vi "Get_modify_set_Protocol2.vi"() -> ()   [LabVIEW 2019]
uses:
  <vilib>/NI VeriStand/Custom Device API/Custom Device Item Ref.ctl
  Addon/Support Libraries/Protocols.lvlibp/TCP/TCP.lvclass
  C:/Dev/niveristand-instrument-addon-custom-device/Source/Addon/Support Libraries/Protocols.lvlibp/Protocol Parent/Protocol Parent.lvclass
  Scripting API/Scripting API.lvlib
  <vilib>/NI VeriStand/Custom Device API/Custom Device API.lvlib
panel:
  out "Instrument Addon Refnum Out":T1=18446744073709551615 format="%.0x"
  out "Error Out":errorcluster
  in  "Error In":errorcluster
  in  "Instrument Addon Refnum In":T1=18446744073709551615 format="%.0x"
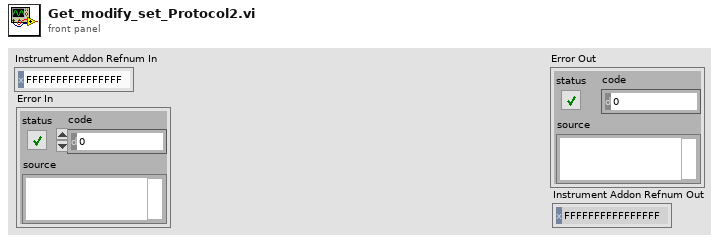
[diagram p1: front panel]
types:
  T1 = typedef "Custom Device API.lvlib/Custom Device Item Ref.ctl" = u64
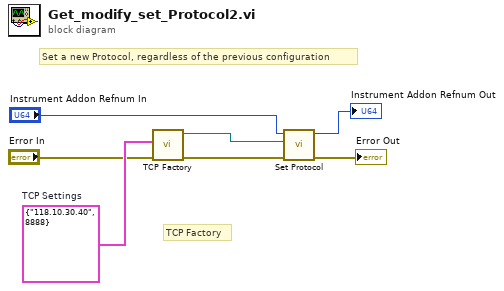
[diagram p0: block diagram]
diagram:
  w5 = cluster{"IP Address":string, "Port":u16} {"IP Address"="118.10.30.40", "Port"=8888}  # TCP Settings
  # "TCP Factory"
  # "Set a new Protocol, regardless of the previous configuration"
  n1 = call "TCP Factory.vi"("error in (no error)"="Error In", "TCP Settings"=w5) -> ("error out"=w2:errorcluster, "TCP out"=w1:refnum<class "TCP.lvclass">)  [unwired: 8 in]
  n2 = call "Set Protocol.vi"("Error In"=w2, "Protocol"=w1, "Instrument Addon Refnum In"="Instrument Addon Refnum In") -> ("Error Out"=→"Error Out":errorcluster, "Instrument Addon Refnum Out"=→"Instrument Addon Refnum Out":T1)  [unwired: 7 in]
